vi "JSON Set.vi"(6 "Pretty Print? (F)":bool, 7 "Behavior (Add or Modify)":T1, 8 "error in (no error)":errorcluster, 9 "Value":variant, 10 "Root Path ([]=Root)":string[](array[string]), 11 "JSON in":string) -> (0 "error out":errorcluster, 2 "Exists?":bool, 3 "JSON out":string)   [LabVIEW 2019, in "labview_json.lvlib"]
doc: "Set an element in the <b>JSON in</b> string by the <b>Value</b> variant specified. \nChange the <b>Behavior</b> to:\n <b>Add or Modify</b> - Add or modify element, arrays resize if necessary, keys are added\n <b>Modify</b> - Modify element only if it exists, arrays do not resize, keys are not added\n <b>Replace</b> - Replace entire element, root paths are exempt\nSpecify the <b>Root Path</b> to the nested object key or array index. \nWhen the <b>Behavior</b> is <b>Replace</b>, nested root path objects or arrays are kept. \n<b>Exists?</b> only returns True if all elements are found. \n<b>Pretty Print?</b> whitespace indents the <b>JSON out</b> string.\nCreated by: Ryan Pacini"
uses:
  labview_json.lvlib
  Element Set Behavior.ctl
  <vilib>/Utility/error.llb/Error Cluster From Error Code.vi
  <vilib>/ErrorRing/Error Ring.xnode
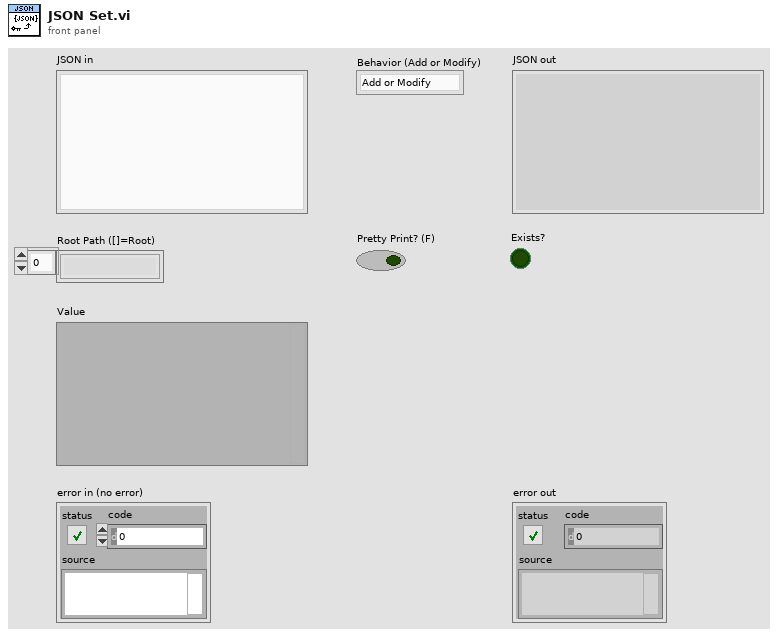
[diagram p1: front panel]
types:
  T1 = typedef "labview_json.lvlib/Element Set Behavior.ctl" = enum8{"Add or Modify", "Modify Only", "Replace"}
  T2 = typedef "labview_json.lvlib/Element.ctl" = cluster{"Key":string, "Type":T3, "Value":variant, "IsRootPath":bool}
  T3 = typedef "labview_json.lvlib/Element Type.ctl" = enum8{"NULL", "OBJECT", "ARRAY", "BOOL", "INT", "UINT", "FLOAT", "STRING"}
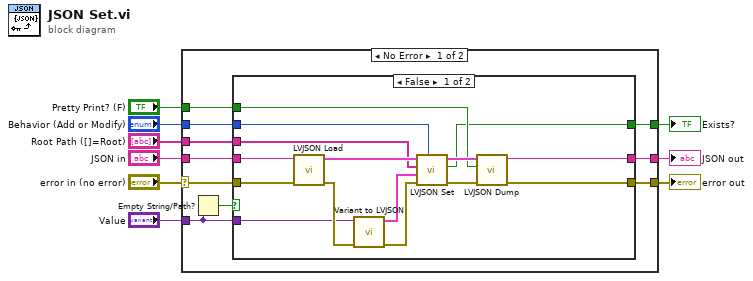
[diagram p0: block diagram]
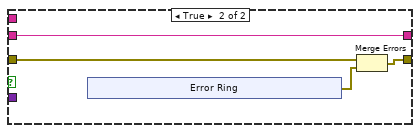
[diagram p2: hidden frame]
diagram:
  n1 = case shown="No Error" "error in (no error)" {
    selector: "error in (no error)" -> [w19 w44]
    tunnel: [w18 w44] -> w8
    tunnel: "JSON in" -> [w17 w43]
    tunnel: [w16 w43] -> w6
    tunnel: "Root Path ([]=Root)" -> [w15 _]
    tunnel: "Value" -> [w11 _]
    tunnel: "Pretty Print? (F)" -> [w14 _]
    tunnel: [w13 _] -> w2
    tunnel: "Behavior (Add or Modify)" -> [w12 _]
    frame No Error {
      n2 = Empty String/Path?(string/path=w11) -> (empty?=w10:bool)
      n3 = case shown="False" w10 {
        tunnel: w19 -> [w34 w37]
        tunnel: [w33 w36] -> w18
        tunnel: w17 -> [w32 w38]
        tunnel: [w31 w38] -> w16
        tunnel: w15 -> [w28 _]
        tunnel: w14 -> [w24 _]
        tunnel: [w23 _] -> w13
        tunnel: w12 -> [w21 _]
        tunnel: w11 -> [w20 _]
        frame False {
          n4 = call "LVJSON Load.vi"("error in (no error)"=w34, "JSON in"=w32) -> ("error out"=w27:errorcluster, "Root Element out"=w30:T2)  [unwired: 8 in]
          n5 = call "Variant to LVJSON.vi"("error in (no error)"=w27, "Variant in"=w20) -> ("error out"=w26:errorcluster, "Element out"=w25:T2)  [unwired: 8 in]
          n6 = call "LVJSON Set.vi"("Behavior (Add or Modify)"=w21, "error in (no error)"=w26, "Element"=w25, "Root Path"=w28, "Root Element in"=w30) -> ("error out"=w22:errorcluster, "Exists?"=w23:bool, "Root Element out"=w29:T2)  [unwired: 4 in]
          n7 = call "LVJSON Dump.vi"("error in (no error)"=w22, "Pretty Print? (F)"=w24, "Root Element in"=w29) -> ("error out"=w33:errorcluster, "JSON out"=w31:string)  [unwired: 6 in, 1 out]
        }
        frame True {
          n8 = xnode "Error Ring"() -> ("error out"=w35:errorcluster)
          n9 = Merge Errors(w37, w35) -> (w36:errorcluster)
        }
      }
    }
    frame Error {
    }
  }
  "error out" <- w8
  "JSON out" <- w6
  "Exists?" <- w2
